vi "GLdrv_RW.vi"(4 "timeout(10s)":u32=10000, 5 "Term(CrLf)":string="\r\n", 6 "Mode(read)":T1=enum."Read", 8 "error in (no error)":errorcluster, 9 "Count(0:[CR+LF])":u32, 10 "data in":string, 11 "Connection ID":T2) -> (0 "error out":errorcluster, 1 "Mode.Ref":T1=enum."Read", 2 "data out":string, 3 "Connection ID Out":T2)   [LabVIEW 2017]
uses:
  ConnectionID.ctl
  GLdrv_RW.ctl
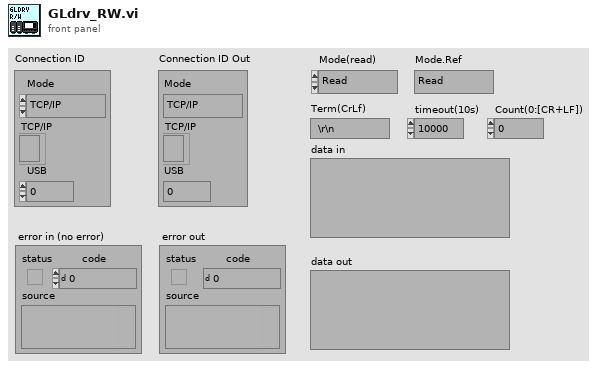
[diagram p1: front panel]
types:
  T1 = typedef "GLdrv_RW.ctl" = enum16{"Auto", "Read", "Write", "Buffer"}
  T2 = typedef "ConnectionID.ctl" = cluster{"Mode":enum16{"TCP/IP", "USB"}, "TCP/IP":refnum<k5>, "USB":i32}
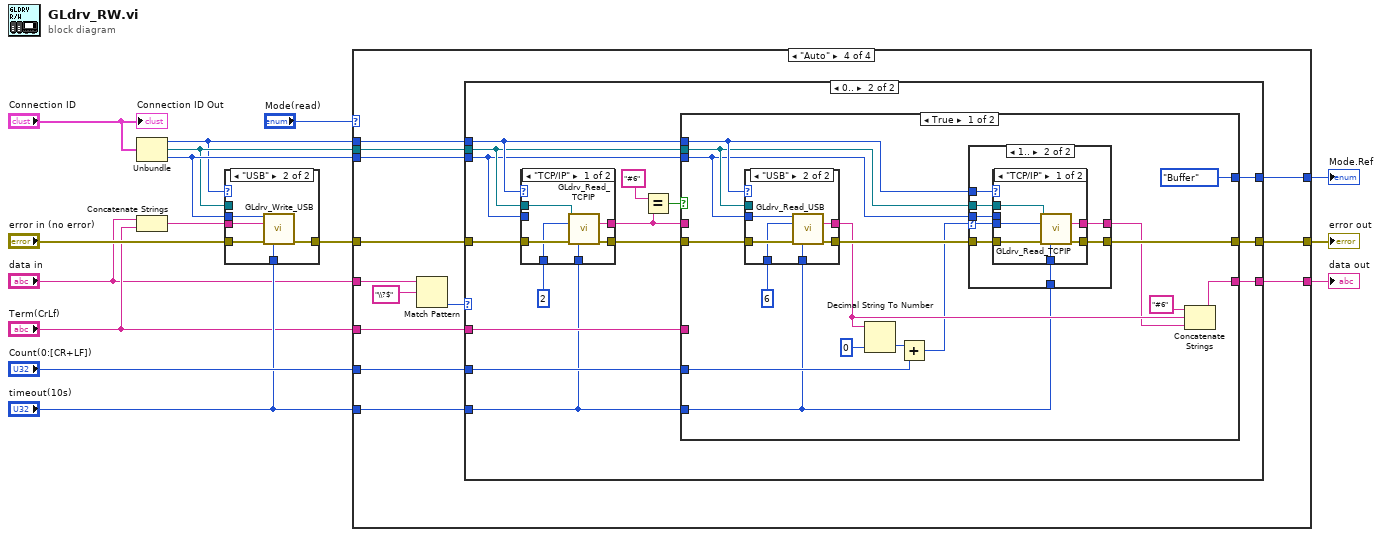
[diagram p0: block diagram]
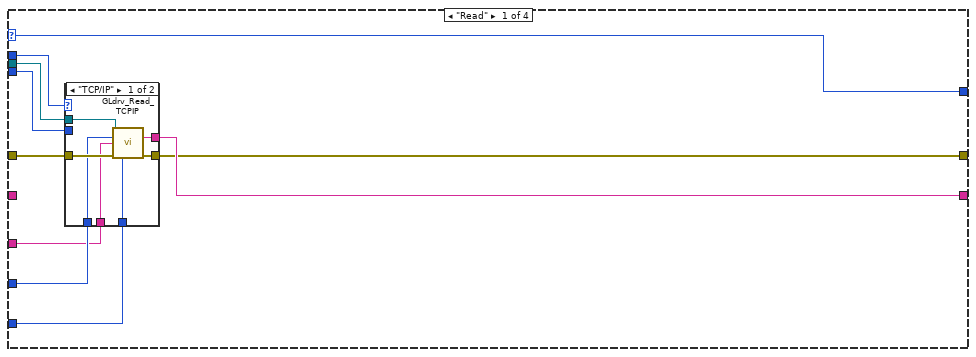
[diagram p2: hidden frame]
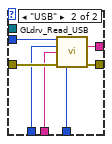
[diagram p3: hidden frame]
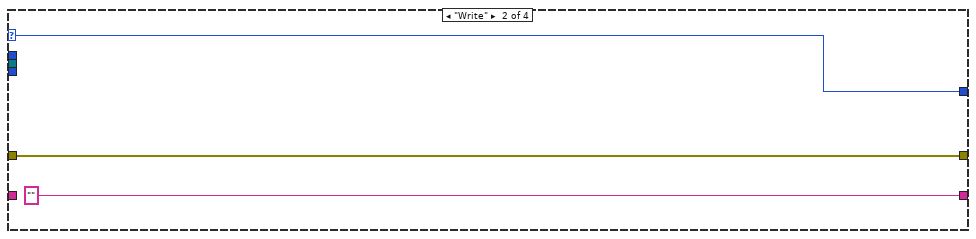
[diagram p4: hidden frame]
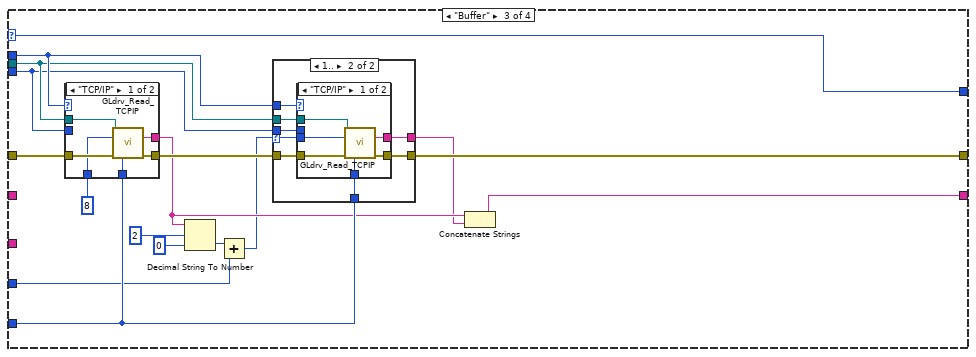
[diagram p5: hidden frame]
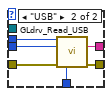
[diagram p7: hidden frame]
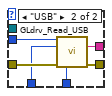
[diagram p8: hidden frame]
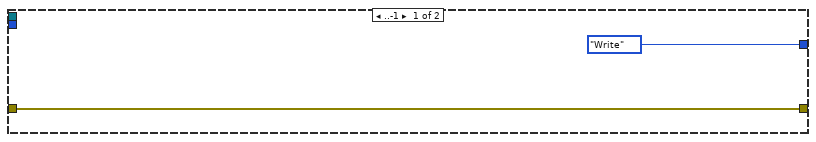
[diagram p9: hidden frame]
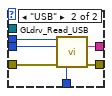
[diagram p11: hidden frame]
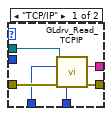
[diagram p12: hidden frame]
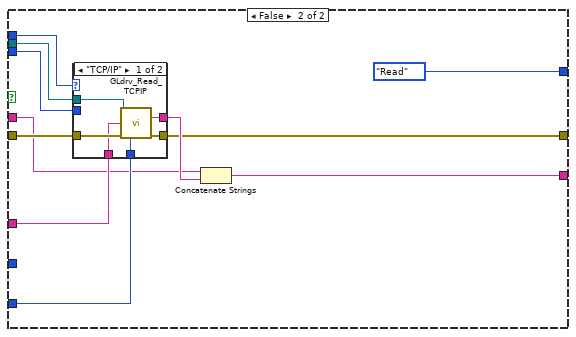
[diagram p13: hidden frame]
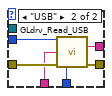
[diagram p14: hidden frame]
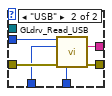
[diagram p15: hidden frame]
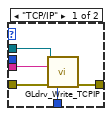
[diagram p16: hidden frame]
diagram:
  n1 = Unbundle("Connection ID") -> ("Mode"=w9:enum16{"TCP/IP", "USB"}, "TCP/IP"=w10:refnum<k5>, "USB"=w11:i32)
  n2 = Concatenate Strings("data in", "Term(CrLf)") -> (w3:string)
  n3 = case shown="\"USB\"" w9 {
    tunnel: w3 -> [w20 w25]
    tunnel: w10 -> [w19 _]
    tunnel: "error in (no error)" -> [w18 w24]
    tunnel: [w17 w23] -> w7
    tunnel: w11 -> [_ w22]
    tunnel: "timeout(10s)" -> [w16 w21]
    frame "TCP/IP" {
      n4 = call "GLdrv_Write_TCPIP.vi"("connection ID"=w19, "data in"=w20, "error in (no error)"=w18, "timeout ms (25000)"=w16) -> ("error out"=w17:errorcluster)  [unwired: 11 out]
    }
    frame "USB" {
      n5 = call "GLdrv_Write_USB.vi"("hDevice"=w22, "lpBuffer"=w25, "error in (no error)"=w24, "dwTimeOut"=w21) -> ("error out"=w23:errorcluster)  [unwired: 11 out]
    }
  }
  n6 = case shown="\"Auto\"" "Mode(read)" {
    selector: "Mode(read)" -> [w26 w50 w54 _]
    tunnel: "Count(0:[CR+LF])" -> [w35 _ w56 w113]
    tunnel: [w34 "" ("lpBuffer") w58 w114] -> w14
    tunnel: [w33 w52 w62 w115] -> w13
    tunnel: w11 -> [w32 _ w64 w110]
    tunnel: w10 -> [w31 _ w65 w111]
    tunnel: w9 -> [w30 _ w66 w112]
    tunnel: w7 -> [w29 w52 w69 w109]
    tunnel: "timeout(10s)" -> [w28 _ w68 w107]
    tunnel: "Term(CrLf)" -> [w27 _ _ w108]
    tunnel: "data in" -> [_ _ _ w106]
    tunnel: [w26 w50 w54 w103] -> w2
    frame "Read" {
      n7 = case shown="\"TCP/IP\"" w30 {
        tunnel: [w39 w46] -> w34
        tunnel: w31 -> [w42 _]
        tunnel: w29 -> [w41 w49]
        tunnel: [w40 w47] -> w33
        tunnel: w32 -> [_ w48]
        tunnel: w28 -> [w38 w45]
        tunnel: w35 -> [w37 w44]
        tunnel: w27 -> [w36 w43]
        frame "TCP/IP" {
          n8 = call "GLdrv_Read_TCPIP.vi"("connection ID"=w42, "Count"=w37, "Term(CrLf)"=w36, "error in (no error)"=w41, "timeout ms"=w38) -> ("data out"=w39:string, "error out"=w40:errorcluster)  [unwired: 9 out]
        }
        frame "USB" {
          n9 = call "GLdrv_Read_USB.vi"("hDevice"=w48, "Count"=w44, "Term(CrLf)"=w43, "error in (no error)"=w49, "dwTimeOut"=w45) -> ("lpBuffer"=w46:string, "error out"=w47:errorcluster)  [unwired: 9 out]
        }
      }
    }
    frame "Write" {
    }
    frame "Buffer" {
      n10 = case shown="\"TCP/IP\"" w66 {
        tunnel: [w93 w99] -> w59
        tunnel: w65 -> [w96 _]
        tunnel: w69 -> [w95 w102]
        tunnel: [w94 w100] -> w63
        tunnel: w64 -> [_ w101]
        tunnel: w68 -> [w92 w98]
        tunnel: u32 8 ("Count(0:[CR+LF])") -> [w91 w97]
        frame "TCP/IP" {
          n11 = call "GLdrv_Read_TCPIP.vi"("connection ID"=w96, "Count"=w91, "error in (no error)"=w95, "timeout ms"=w92) -> ("data out"=w93:string, "error out"=w94:errorcluster)  [unwired: 1 in, 9 out]
        }
        frame "USB" {
          n12 = call "GLdrv_Read_USB.vi"("hDevice"=w101, "Count"=w97, "error in (no error)"=w102, "dwTimeOut"=w98) -> ("lpBuffer"=w99:string, "error out"=w100:errorcluster)  [unwired: 1 in, 9 out]
        }
      }
      n13 = Decimal String To Number(string=w59, offset=2, default (0L)=u32 0 ("default (0 I32)")) -> (number=w61:u32)  [unwired: 1 out]
      n14 = Add(x=w61, y=w56) -> (x+y=w53:u32)
      n15 = case shown="1.." w53 {
        selector: w53 -> [_ w71]
        tunnel: w68 -> [_ w78]
        tunnel: w66 -> [_ w77]
        tunnel: w65 -> [_ w76]
        tunnel: w64 -> [_ w75]
        tunnel: w63 -> [w70 w74]
        tunnel: [w70 w73] -> w62
        tunnel: [_ w72] -> w57
        frame ..0 {
        }
        frame 1.. {
          n16 = case shown="\"TCP/IP\"" w77 {
            tunnel: [w81 w87] -> w72
            tunnel: w76 -> [w84 _]
            tunnel: w74 -> [w83 w90]
            tunnel: [w82 w88] -> w73
            tunnel: w75 -> [_ w89]
            tunnel: w78 -> [w80 w86]
            tunnel: w71 -> [w79 w85]
            frame "TCP/IP" {
              n17 = call "GLdrv_Read_TCPIP.vi"("connection ID"=w84, "Count"=w79, "error in (no error)"=w83, "timeout ms"=w80) -> ("data out"=w81:string, "error out"=w82:errorcluster)  [unwired: 1 in, 9 out]
            }
            frame "USB" {
              n18 = call "GLdrv_Read_USB.vi"("hDevice"=w89, "Count"=w85, "error in (no error)"=w90, "dwTimeOut"=w86) -> ("lpBuffer"=w87:string, "error out"=w88:errorcluster)  [unwired: 1 in, 9 out]
            }
          }
        }
      }
      n19 = Concatenate Strings(w59, w57) -> (w58:string)
    }
    frame "Auto" {
      n20 = Match Pattern(string=w106, regular expression="\\?$") -> (offset past match=w104:i32)  [unwired: 1 in, 3 out]
      n21 = case shown="0.." w104 {
        tunnel: [w117 w132] -> w115
        tunnel: [_ w131] -> w114
        tunnel: w113 -> [_ w130]
        tunnel: w112 -> [_ w128]
        tunnel: w111 -> [_ w127]
        tunnel: w110 -> [_ w126]
        tunnel: w109 -> [w117 w125]
        tunnel: w108 -> [_ w123]
        tunnel: w107 -> [_ w122]
        tunnel: [GLdrv_RW."Write" ("Mode.Ref") w118] -> w103
        frame ..-1 {
        }
        frame 0.. {
          n22 = case shown="\"TCP/IP\"" w128 {
            tunnel: [w208 w214] -> w119
            tunnel: w127 -> [w211 _]
            tunnel: w125 -> [w210 w217]
            tunnel: [w209 w215] -> w124
            tunnel: w126 -> [_ w216]
            tunnel: w122 -> [w207 w213]
            tunnel: u32 2 ("Count(0:[CR+LF])") -> [w206 w212]
            frame "TCP/IP" {
              n23 = call "GLdrv_Read_TCPIP.vi"("connection ID"=w211, "Count"=w206, "error in (no error)"=w210, "timeout ms"=w207) -> ("data out"=w208:string, "error out"=w209:errorcluster)  [unwired: 1 in, 9 out]
            }
            frame "USB" {
              n24 = call "GLdrv_Read_USB.vi"("hDevice"=w216, "Count"=w212, "error in (no error)"=w217, "dwTimeOut"=w213) -> ("lpBuffer"=w214:string, "error out"=w215:errorcluster)  [unwired: 1 in, 9 out]
            }
          }
          n25 = Equal?(x="#6", y=w119) -> (x = y?=w120:bool)
          n26 = case shown="TRUE" w120 {
            tunnel: [w147 w184] -> w132
            tunnel: [w144 w192] -> w131
            tunnel: w130 -> [w142 _]
            tunnel: w128 -> [w140 w191]
            tunnel: w127 -> [w139 w190]
            tunnel: w126 -> [w138 w189]
            tunnel: w124 -> [w137 w188]
            tunnel: w123 -> [_ w187]
            tunnel: w122 -> [w136 w186]
            tunnel: w119 -> [_ w185]
            tunnel: [GLdrv_RW."Buffer" ("Mode.Ref") GLdrv_RW."Read" ("Mode.Ref")] -> w118
            frame True {
              n27 = case shown="\"USB\"" w140 {
                tunnel: [w173 w179] -> w145
                tunnel: w139 -> [w176 _]
                tunnel: w137 -> [w175 w182]
                tunnel: [w174 w180] -> w148
                tunnel: w138 -> [_ w181]
                tunnel: w136 -> [w172 w178]
                tunnel: u32 6 ("Count(0:[CR+LF])") -> [w171 w177]
                frame "TCP/IP" {
                  n28 = call "GLdrv_Read_TCPIP.vi"("connection ID"=w176, "Count"=w171, "error in (no error)"=w175, "timeout ms"=w172) -> ("data out"=w173:string, "error out"=w174:errorcluster)  [unwired: 1 in, 9 out]
                }
                frame "USB" {
                  n29 = call "GLdrv_Read_USB.vi"("hDevice"=w181, "Count"=w177, "error in (no error)"=w182, "dwTimeOut"=w178) -> ("lpBuffer"=w179:string, "error out"=w180:errorcluster)  [unwired: 1 in, 9 out]
                }
              }
              n30 = Decimal String To Number(string=w145, default (0L)=u32 0 ("default (0 I32)")) -> (number=w146:u32)  [unwired: 1 in, 1 out]
              n31 = Add(x=w146, y=w142) -> (x+y=w133:u32)
              n32 = case shown="1.." w133 {
                selector: w133 -> [_ w151]
                tunnel: w148 -> [w150 w158]
                tunnel: [w150 w157] -> w147
                tunnel: [_ w156] -> w143
                tunnel: w140 -> [_ w155]
                tunnel: w139 -> [_ w154]
                tunnel: w138 -> [_ w153]
                tunnel: w136 -> [_ w152]
                frame ..0 {
                }
                frame 1.. {
                  n33 = case shown="\"TCP/IP\"" w155 {
                    tunnel: [w161 w167] -> w156
                    tunnel: w154 -> [w164 _]
                    tunnel: w158 -> [w163 w170]
                    tunnel: [w162 w168] -> w157
                    tunnel: w153 -> [_ w169]
                    tunnel: w152 -> [w160 w166]
                    tunnel: w151 -> [w159 w165]
                    frame "TCP/IP" {
                      n34 = call "GLdrv_Read_TCPIP.vi"("connection ID"=w164, "Count"=w159, "error in (no error)"=w163, "timeout ms"=w160) -> ("data out"=w161:string, "error out"=w162:errorcluster)  [unwired: 1 in, 9 out]
                    }
                    frame "USB" {
                      n35 = call "GLdrv_Read_USB.vi"("hDevice"=w169, "Count"=w165, "error in (no error)"=w170, "dwTimeOut"=w166) -> ("lpBuffer"=w167:string, "error out"=w168:errorcluster)  [unwired: 1 in, 9 out]
                    }
                  }
                }
              }
              n36 = Concatenate Strings("#6" ("x"), w145, w143) -> (w144:string)
            }
            frame False {
              n37 = case shown="\"TCP/IP\"" w191 {
                tunnel: [w196 w202] -> w193
                tunnel: w190 -> [w199 _]
                tunnel: w188 -> [w198 w205]
                tunnel: [w197 w203] -> w184
                tunnel: w189 -> [_ w204]
                tunnel: w186 -> [w195 w201]
                tunnel: w187 -> [w194 w200]
                frame "TCP/IP" {
                  n38 = call "GLdrv_Read_TCPIP.vi"("connection ID"=w199, "Term(CrLf)"=w194, "error in (no error)"=w198, "timeout ms"=w195) -> ("data out"=w196:string, "error out"=w197:errorcluster)  [unwired: 1 in, 9 out]
                }
                frame "USB" {
                  n39 = call "GLdrv_Read_USB.vi"("hDevice"=w204, "Term(CrLf)"=w200, "error in (no error)"=w205, "dwTimeOut"=w201) -> ("lpBuffer"=w202:string, "error out"=w203:errorcluster)  [unwired: 1 in, 9 out]
                }
              }
              n40 = Concatenate Strings(w185, w193) -> (w192:string)
            }
          }
        }
      }
    }
  }
  "data out" <- w14
  "error out" <- w13
  "Mode.Ref" <- w2
  "Connection ID Out" <- "Connection ID"
